vi "Logging_2.vi"(2 "Voltage Command":dbl, 6 "Setpoint":dbl, 8 "error in":errorcluster, 9 "Filename":path=path "C:/1. Rocket Research Project/CollectedData/Plots/TestingData.lvm", 10 "Enable":bool=TRUE, 11 "output cluster":T1) -> (0 "error out":errorcluster)   [LabVIEW 2022 SP3]
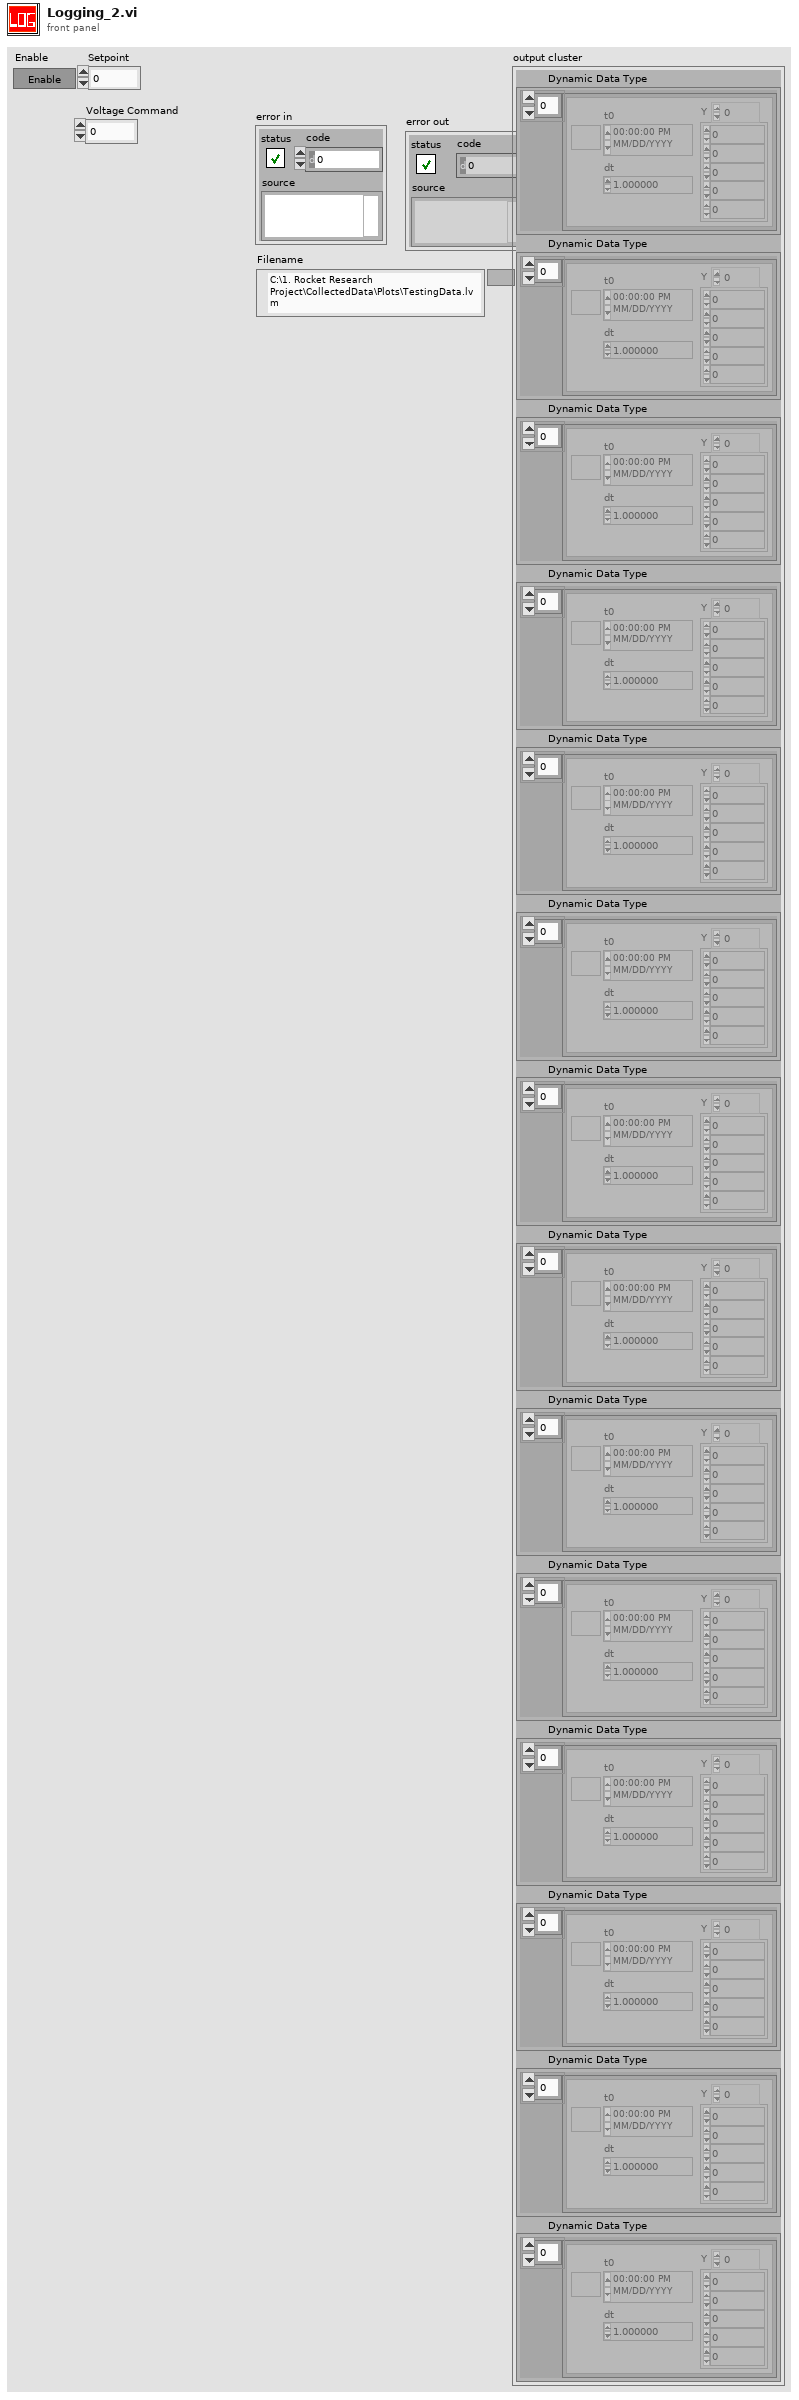
[diagram p1: front panel]
types:
  T1 = cluster{"Dynamic Data Type":dynamicdata, "Dynamic Data Type":dynamicdata, "Dynamic Data Type":dynamicdata, "Dynamic Data Type":dynamicdata, "Dynamic Data Type":dynamicdata, "Dynamic Data Type":dynamicdata, "Dynamic Data Type":dynamicdata, "Dynamic Data Type":dynamicdata, "Dynamic Data Type":dynamicdata, "Dynamic Data Type":dynamicdata, "Dynamic Data Type":dynamicdata, "Dynamic Data Type":dynamicdata, "Dynamic Data Type":dynamicdata, "Dynamic Data Type":dynamicdata}
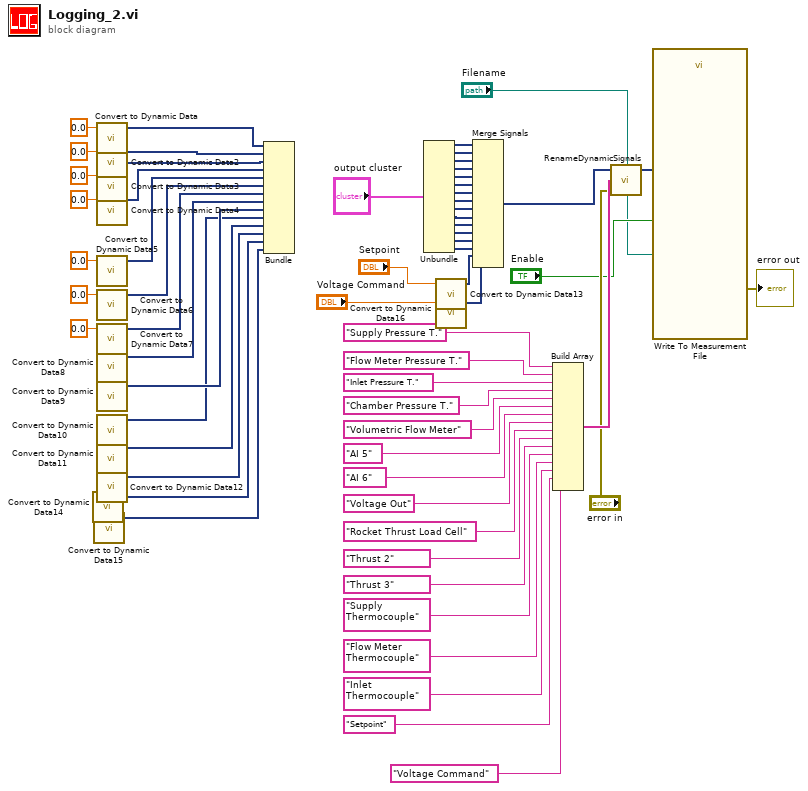
[diagram p0: block diagram]
diagram:
  n1 = call "Convert to Dynamic Data14"() -> ("Dynamic Data Type"=w12:dynamicdata)  [unwired: 4 in]
  n2 = call "Convert to Dynamic Data15"() -> ("Dynamic Data Type"=w11:dynamicdata)  [unwired: 4 in]
  n3 = call "Convert to Dynamic Data"("Double"=0.0) -> ("Dynamic Data Type"=w60:dynamicdata)  [unwired: 3 in]
  n4 = call "Convert to Dynamic Data2"("Double"=0.0) -> ("Dynamic Data Type"=w59:dynamicdata)  [unwired: 3 in]
  n5 = call "Convert to Dynamic Data3"("Double"=0.0) -> ("Dynamic Data Type"=w53:dynamicdata)  [unwired: 3 in]
  n6 = call "Convert to Dynamic Data4"("Double"=0.0) -> ("Dynamic Data Type"=w52:dynamicdata)  [unwired: 3 in]
  n7 = call "Convert to Dynamic Data5"("Double"=0.0) -> ("Dynamic Data Type"=w51:dynamicdata)  [unwired: 3 in]
  n8 = call "Convert to Dynamic Data6"("Double"=0.0) -> ("Dynamic Data Type"=w50:dynamicdata)  [unwired: 3 in]
  n9 = call "Convert to Dynamic Data7"("Double"=0.0) -> ("Dynamic Data Type"=w49:dynamicdata)  [unwired: 3 in]
  n10 = call "Convert to Dynamic Data8"() -> ("Dynamic Data Type"=w48:dynamicdata)  [unwired: 4 in]
  n11 = call "Convert to Dynamic Data9"() -> ("Dynamic Data Type"=w47:dynamicdata)  [unwired: 4 in]
  n12 = call "Convert to Dynamic Data10"() -> ("Dynamic Data Type"=w46:dynamicdata)  [unwired: 4 in]
  n13 = call "Convert to Dynamic Data11"() -> ("Dynamic Data Type"=w45:dynamicdata)  [unwired: 4 in]
  n14 = call "Convert to Dynamic Data12"() -> ("Dynamic Data Type"=w44:dynamicdata)  [unwired: 4 in]
  n15 = Bundle("Dynamic Data Type"=w60, "Dynamic Data Type"=w59, "Dynamic Data Type"=w53, "Dynamic Data Type"=w52, "Dynamic Data Type"=w51, "Dynamic Data Type"=w50, "Dynamic Data Type"=w49, "Dynamic Data Type"=w48, "Dynamic Data Type"=w47, "Dynamic Data Type"=w46, "Dynamic Data Type"=w45, "Dynamic Data Type"=w44, "Dynamic Data Type"=w12, "Dynamic Data Type"=w11) -> ()  [unwired: 1 in, 1 out]
  n16 = Unbundle("output cluster") -> ("Dynamic Data Type"=w32:dynamicdata, "Dynamic Data Type"=w33:dynamicdata, "Dynamic Data Type"=w34:dynamicdata, "Dynamic Data Type"=w35:dynamicdata, "Dynamic Data Type"=w36:dynamicdata, "Dynamic Data Type"=w37:dynamicdata, "Dynamic Data Type"=w38:dynamicdata, "Dynamic Data Type"=w39:dynamicdata, "Dynamic Data Type"=w40:dynamicdata, "Dynamic Data Type"=w41:dynamicdata, "Dynamic Data Type"=w42:dynamicdata, "Dynamic Data Type"=w43:dynamicdata, "Dynamic Data Type"=w8:dynamicdata, "Dynamic Data Type"=w7:dynamicdata)
  n17 = call "Convert to Dynamic Data13"("Double"="Setpoint") -> ("Dynamic Data Type"=w10:dynamicdata)  [unwired: 3 in]
  n18 = call "Convert to Dynamic Data16"("Double"="Voltage Command") -> ("Dynamic Data Type"=w3:dynamicdata)  [unwired: 3 in]
  n19 = Merge Signals(w32, w33, w34, w35, w36, w37, w38, w39, w40, w41, w42, w43, w8, w7, w10, w3) -> (w31:dynamicdata)
  n20 = Build Array("Supply Pressure T.", "Flow Meter Pressure T.", "Inlet Pressure T.", "Chamber Pressure T.", "Volumetric Flow Meter", "AI 5", "AI 6", "Voltage Out" ("element"), "Rocket Thrust Load Cell", "Thrust 2", "Thrust 3", "Supply Thermocouple", "Flow Meter Thermocouple", "Inlet Thermocouple", "Setpoint" ("element"), "Voltage Command" ("element")) -> (w18:string[])
  n21 = call "RenameDynamicSignals.vi"("error in"="error in", "New Signal Names"=w18, "Dynamic Data In"=w31) -> ("Dynamic Data Out"=w63:dynamicdata)  [unwired: 1 in, 1 out]
  n22 = call "Write To Measurement File"("Signals"=w63, "Enable"="Enable", "Filename"="Filename") -> ("error out"=→"error out":errorcluster)  [unwired: 14 in, 2 out]
